vi "Getevrything.vi"(9 "Col":i32, 10 "Row":i32, 11 "Array Dead Or Allive":u32[][](array[numeric])) -> (2 "Array":u32[][][](array[numeric]), 3 "element":u32)   [LabVIEW 2013]
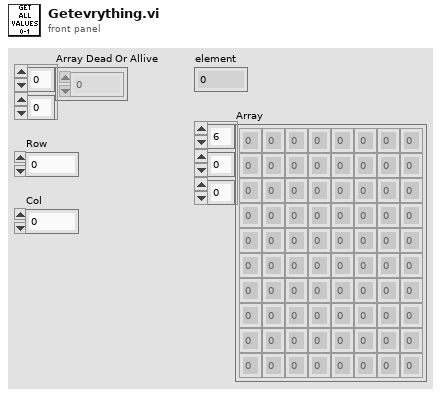
[diagram p1: front panel]
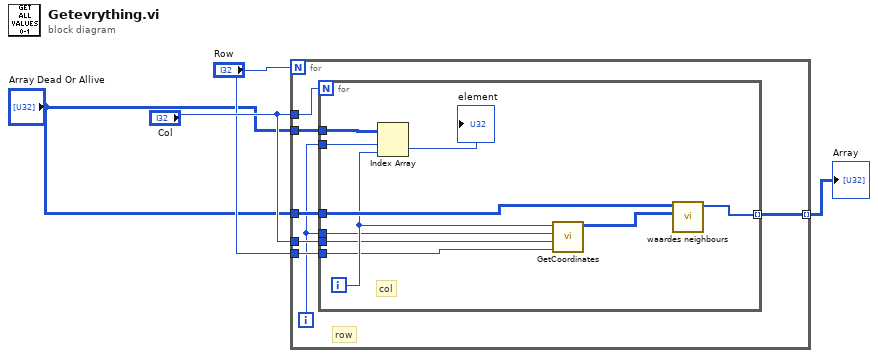
[diagram p0: block diagram]
diagram:
  n1 = for {
    N: "Row" -> [_]
    tunnel: "Col" -> [w11]
    tunnel: "Array Dead Or Allive" -> [w10]
    tunnel: "Col" -> [w9]
    tunnel: "Row" -> [w8]
    tunnel: "Array Dead Or Allive" -> [w7]
    tunnel: [w6] -> w2 mode=indexing
    i -> [w5]
    # "row"
    n2 = for {
      N: w11 -> [_]
      tunnel: w10 -> [w21]
      tunnel: w5 -> [w20]
      tunnel: w9 -> [w15]
      tunnel: w8 -> [w14]
      tunnel: w7 -> [w18]
      tunnel: [w12] -> w6 mode=indexing
      tunnel: w5 -> [w16]
      i -> [w17]
      # "col"
      n3 = Index Array(array=w21, index (row)=w20, index (col)=w17) -> (element=→"element":u32)
      n4 = call "GetCoordinates.vi"("# row"=w14, "# col"=w15, "Row"=w16, "Col"=w17) -> ("ArrayNeighbours"=w13:i32[][])  [unwired: 5 in, 1 out]
      n5 = call "waardes neighbours.vi"("ArrayNeighbours"=w13, "Array Dead Or Allive"=w18) -> ("Array"=w12:u32[])  [unwired: 9 in]
    }
  }
  "Array" <- w2
